vi "buildArrayex1.vi"() -> ()   [LabVIEW 2020]
panel:
  out "subarray":dbl[](array[numeric])
  in  "index":i32
  out "index element indicator":dbl
  out "size(s)":i32[](array[numeric])
  out "appended array 2":dbl[][](array[numeric])
  out "appended array":dbl[](array[numeric])
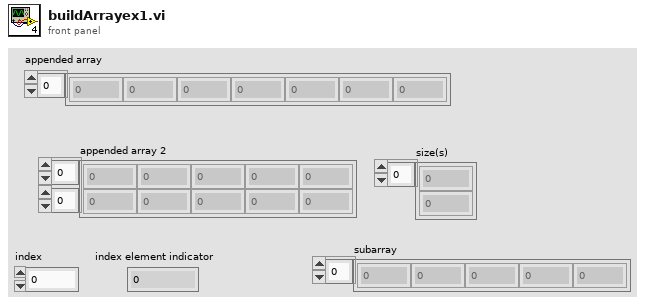
[diagram p1: front panel]
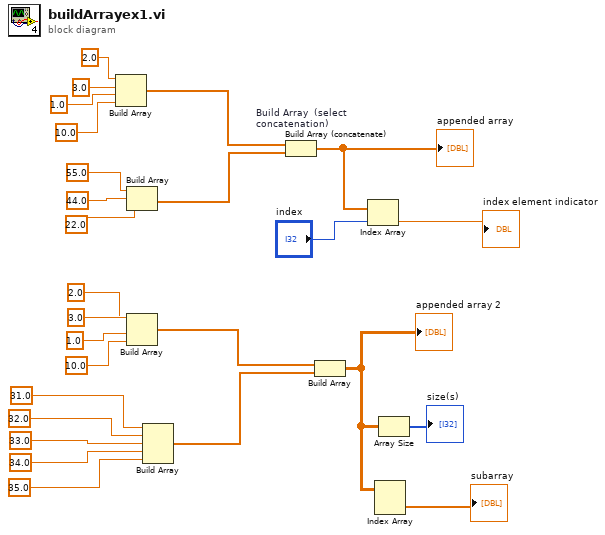
[diagram p0: block diagram]
diagram:
  n1 = Build Array(2.0 ("element"), 3.0 ("element"), 1.0 ("element"), 10.0 ("element")) -> (w22:dbl[])
  n2 = Build Array(55.0 ("element"), 44.0 ("element"), 22.0 ("element")) -> (w21:dbl[])
  n3 = Build Array(2.0 ("element"), 3.0 ("element"), 1.0 ("element"), 10.0 ("element")) -> (w13:dbl[])
  n4 = Build Array(31.0 ("element"), 32.0 ("element"), 33.0 ("element"), 34.0 ("element"), 35.0 ("element")) -> (w7:dbl[])
  n5 = Build Array (concatenate) "Build Array  (select  concatenation)"(w22, w21) -> (w5:dbl[])
  "appended array" <- w5
  n6 = Build Array "Build Array"(w13, w7) -> (w2:dbl[][])
  "appended array 2" <- w2
  n7 = Index Array "Index Array"(array=w5, index="index") -> (element=→"index element indicator":dbl)
  n8 = Index Array(array=w2) -> (element=→"subarray":dbl[])  [unwired: 2 in]
  n9 = Array Size(array=w2) -> (size(s)=→"size(s)":i32[])
